vi "UpDown_Counter.vi"(0 "up":bool, 1 "initial":i32, 3 "down":bool, 4 "reset":bool) -> (5 "count":i32)   [LabVIEW 2016]
doc: "Help by FRC Team 836 - The RoboBees\n\nDescription:\nThis VI will maintain an integer COUNT, incremented by rising edges of UP and decremented by rising edges of DOWN.\nSimultaneous UP and DOWN commands result in no count change, since this is an ambiguous command.\n\nInputs:\nINITIAL - Initial value of COUNT and also value of COUNT upon RESET command\nRESET - Boolean command, COUNT is reset to INITIAL on rising edge, and suspends counting while True. \n Normal operation resumes on falling edge\nUP - Boolean up count signal, operates on rising edge\nDOWN - Boolean down count signal, operates on rising edge\n\nOutputs:\nCOUNT - Outputs and holds current count value"
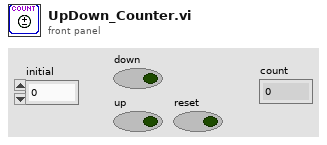
[diagram p1: front panel]
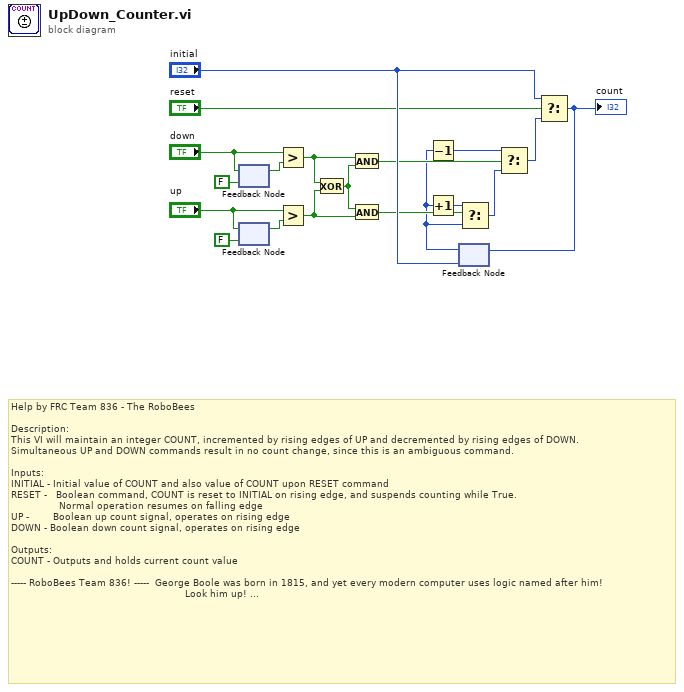
[diagram p0: block diagram]
diagram:
  # "Help by FRC Team 836 - The RoboBees\n\nDescription:\nThis VI will maintain an integer COUNT, incremented by rising edges of UP and decremented by rising edges of DOWN.\nSimultaneous UP and DOWN commands result in no count change, since this is an ambiguous command.\n\nInputs:\nINITIAL - Initial value of COUNT and also value of COUNT upon RESET command\nRESET -   Boolean command, COUNT is reset to INITIAL on rising edge, and suspends counting while True.  \n                Normal operation resumes on falling edge\nUP -        Boolean up count signal, operates on rising edge\nDOWN - Boolean down count signal, operates on rising edge\n\nOutputs:\nCOUNT - Outputs and holds current count value\n\n----- RoboBees Team 836! -----  George Boole was born in 1815, and yet every modern computer uses logic named after him!\n                                                          Look him up! ..."
  n1 = feedback-in #1("down") -> ()
  n2 = feedback #1(FALSE ("down")) -> (w14:bool)
  n3 = feedback #2(FALSE ("down")) -> (w11:bool)
  n4 = feedback-in #2("up") -> ()
  n5 = Greater?(x="down", y=w14) -> (0:w9:bool)
  n6 = Greater?(x="up", y=w11) -> (0:w7:bool)
  n7 = Exclusive Or(1:w7, 2:w9) -> (0:w5:bool)
  n8 = And(x=w9, y=w5) -> (x .and. y?=w8:bool)
  n9 = And(x=w5, y=w7) -> (x .and. y?=w6:bool)
  n10 = feedback #3("initial") -> (w3:i32)
  n11 = Decrement(x=w3) -> (x-1=w18:i32)
  n12 = Increment(x=w3) -> (x+1=w17:i32)
  n13 = Select(t=w17, s=w6, f=w3) -> (s? t:f=w19:i32)
  n14 = Select(t=w18, s=w8, f=w19) -> (s? t:f=w2:i32)
  n15 = Select(t="initial", s="reset", f=w2) -> (s? t:f=w1:i32)
  "count" <- w1
  n16 = feedback-in #3(w1) -> ()
